vi "Read Bus Monitor Entries.vi"(7 "number of entries":i32=100, 8 "error in":errorcluster, 11 "module handle":u32) -> (0 "error out":errorcluster, 2 "Queue Entries":T1[](array[typedef]), 3 "module handle out":u32)   [LabVIEW 2020, in "AIM MIL-STD-1553 Hardware API.lvlib"]
uses:
  AIM MIL-STD-1553 Hardware API.lvlib
  Shortened Queue Entry.ctl
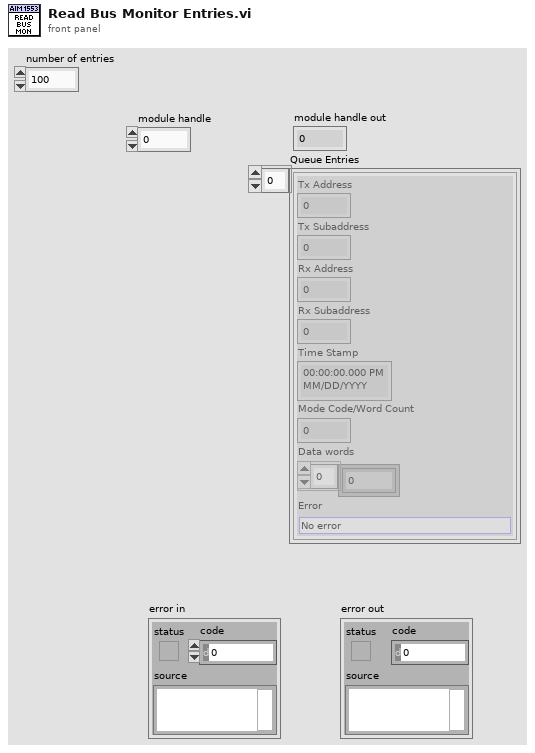
[diagram p1: front panel]
types:
  T1 = typedef "AIM MIL-STD-1553 Hardware API.lvlib/Shortened Queue Entry.ctl" = cluster{"Tx Address":u8, "Tx Subaddress":u8, "Rx Address":u8, "Rx Subaddress":u8, "Time Stamp":timestamp, "Mode Code/Word Count":u8, "Data words":u16[], "Error ":enum16{"No error", "Terminal no response error", "Manchester coding error", "High bit count error", "Low bit count error", "Parity error", "Inverted sync error", "Interw ord gap error", "Transmission on both MILbus channels", "Reserved mode code error", "Early response or gap too short", "ME bit set in status word", "Status word exception error", "High wordcount error", "Low wordcount error", "Illegal command word"}}
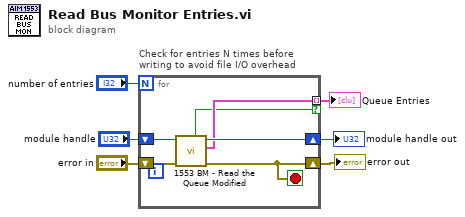
[diagram p0: block diagram]
diagram:
  n1 = for "Check for entries N times before \nwriting to avoid file I/O overhead" {
    N: "number of entries" -> [_]
    shift-right: [w10] -> w4
    shift-left: "module handle" -> [w12]
    shift-right: [w9] -> w3
    shift-left: "error in" -> [w11]
    tunnel: [w8] -> w1 mode=indexing if=w7
    stop <- w9 stop-if-true
    n2 = call "1553 BM - Read the Queue Modified.vi"("Error In (none)"=w11, "Module Handle"=w12) -> ("Error Out"=w9:errorcluster, "Short Queue Entry"=w8:T1, "ModuleHandle Out"=w10:u32, "Queue Entry full"=w7:bool)  [unwired: 6 in]
  }
  "error out" <- w3
  "module handle out" <- w4
  "Queue Entries" <- w1
